vi "Excel.vi"() -> ()   [LabVIEW 2017]
uses:
  <vilib>/addons/_office/excel.llb/Excel Get Data ([str]).vi
  <vilib>/Utility/NIReport.llb/NI_report.lvclass
  <vilib>/Utility/NIReport.llb/Excel/NI_Excel.lvclass
  <vilib>/addons/_office/NI_ReportGenerationToolkit.lvlib
panel:
  out "data":string[][](array[string])
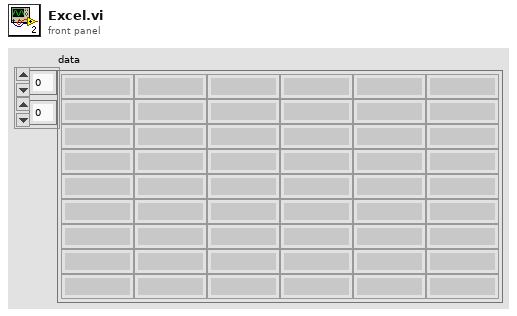
[diagram p1: front panel]
types:
  T1 = enum16{"Standard Report", "HTML", "Word", "Excel"}
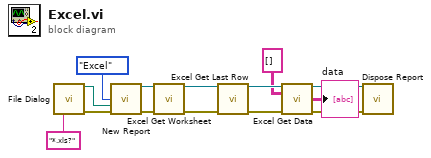
[diagram p0: block diagram]
diagram:
  n1 = call "File Dialog"("pattern (all files)"="*.xls?") -> ("selected path"=w12:path, "error out"=w13:errorcluster)  [unwired: 11 in, 2 out]
  n2 = call <vilib>:"New Report.vi"("report type"=T1."Excel", "template (empty)"=w12, "error in (no error)"=w13) -> ("report out"=w9:refnum<class "NI_report.lvclass">, "error out"=w10:errorcluster)  [unwired: 11 in]
  n3 = call <vilib>:"Excel Get Worksheet.vi"("report in"=w9, "error in (no error)"=w10) -> ("report out"=w7:refnum<class "NI_report.lvclass">, "error out"=w8:errorcluster)  [unwired: 12 in]
  n4 = call <vilib>:"Excel Get Last Row.vi"("report in"=w7, "error in (no error)"=w8) -> ("report out"=w6:refnum<class "NI_report.lvclass">, "error out"=w5:errorcluster)  [unwired: 11 in, 1 out]
  n5 = call-poly <vilib>:"Excel Get Data.vi"("report in"=w6, "data type"=string[][] [], "error in (no error)"=w5) -> ("report out"=w2:refnum<class "NI_report.lvclass">, "data"=→"data":string[][], "error out"=w3:errorcluster)  [unwired: 10 in]
  n6 = call-dynamic "Dispose Report.vi"("report in"=w2, "error in (no error)"=w3) -> ()  [unwired: 13 in, 1 out]
